vi "testSendCmdStatusServersAandB.vi"(8 "error in (no error)":errorcluster) -> (0 "error out":errorcluster)   [LabVIEW 2018]
doc: "Test the sendCmdStatus.vi in TCP/IP servers A and B."
uses:
  src/TcpServer/TcpServer.lvclass
  src/TcpServer/TcpServer.lvclass/TcpServer.ctl
  src/TcpServerCmd/TcpServerCmd.lvclass/TcpServerCmd.ctl
  <vilib>/addons/_JKI Toolkits/Caraya/classes/Assert/Assert Equal Value_Variant.vi
  src/TcpServerCmd/TcpServerCmd.lvclass
  <vilib>/addons/_JKI Toolkits/Caraya/classes/Test/Test.lvclass
  <vilib>/addons/_JKI Toolkits/Caraya/classes/Assert/Assert.lvclass
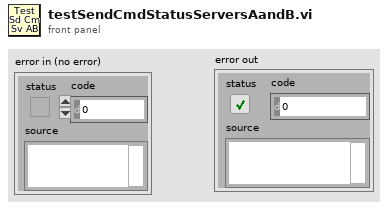
[diagram p1: front panel]
types:
  T1 = typedef "TcpServerCmd.lvclass/userEventTypeDef.ctl" = cluster{"CmdRead":refnum<user-event>, "CmdWrite":refnum<user-event>, "EvtRead":refnum<user-event>, "EvtWrite":refnum<user-event>}
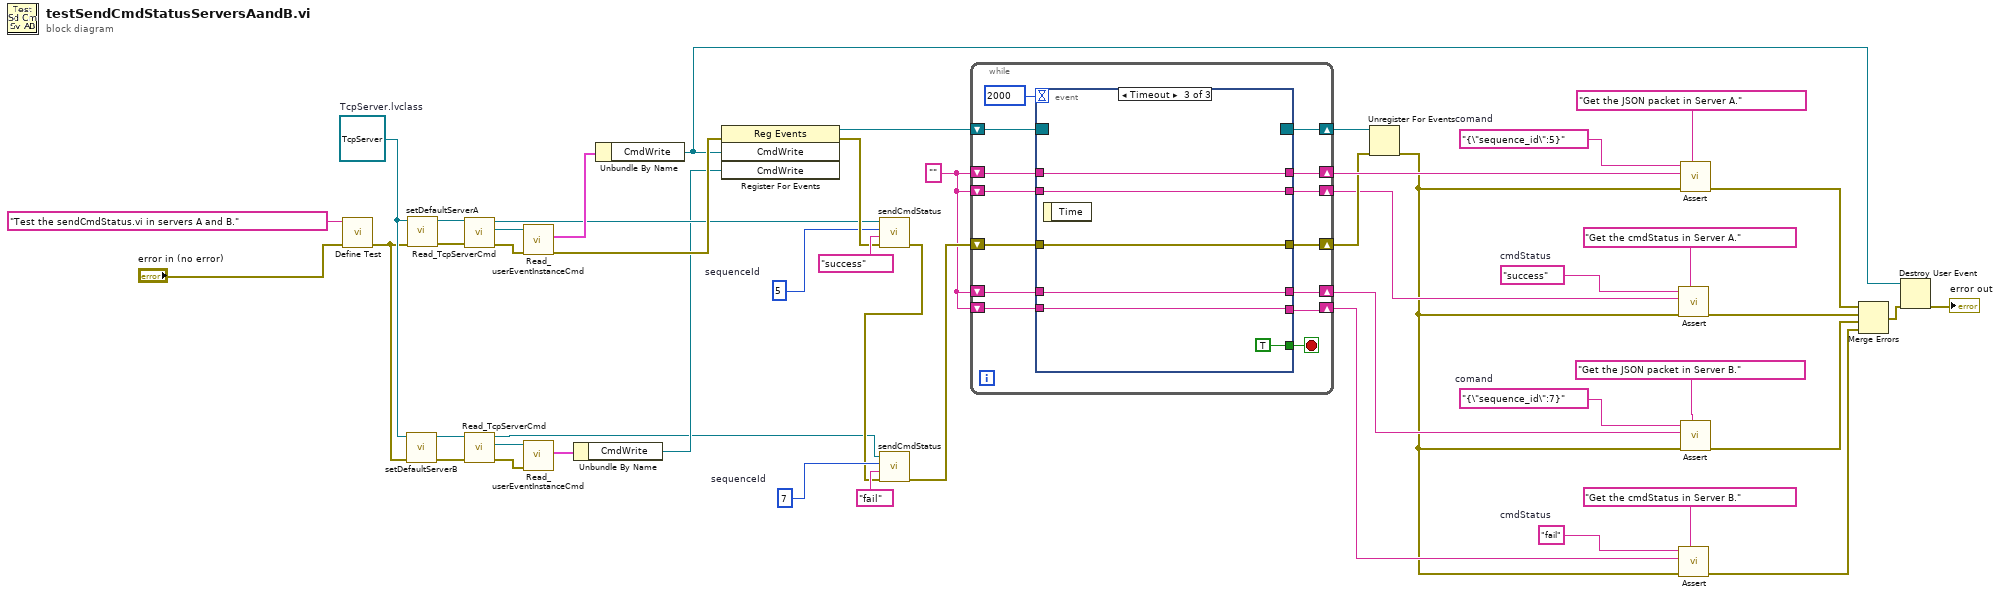
[diagram p0: block diagram]
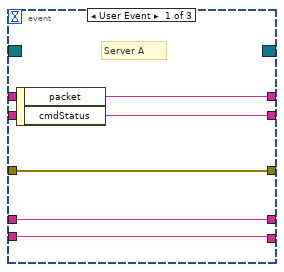
[diagram p2: hidden frame]
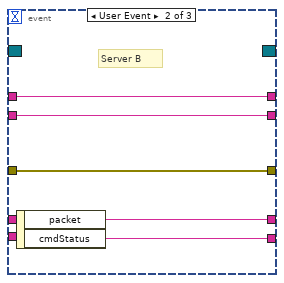
[diagram p3: hidden frame]
diagram:
  w6 = "" ("packet")
  w9 = "fail"  # cmdStatus
  w8 = "{\"sequence_id\":7}"  # comand
  w15 = 7  # sequenceId
  w26 = 5  # sequenceId
  w33 = "success"  # cmdStatus
  w42 = "{\"sequence_id\":5}"  # comand
  w23 = refnum<class "TcpServer.lvclass"> refnum  # TcpServer.lvclass
  n1 = call <vilib>:"Define Test.vi"("error in (no error)"="error in (no error)", "Label (VI Title)"="Test the sendCmdStatus.vi in servers A and B.") -> ("error out"=w22:errorcluster)  [unwired: 9 in]
  n2 = call "setDefaultServerB.vi"("error in (no error)"=w22, "TcpServer.lvclass"=w23) -> ("error out"=w18:errorcluster, "tcpServer out"=w19:refnum<class "TcpServer.lvclass">)  [unwired: 8 in]
  n3 = call "setDefaultServerA.vi"("error in (no error)"=w22, "TcpServer.lvclass"=w23) -> ("error out"=w25:errorcluster, "tcpServer out"=w24:refnum<class "TcpServer.lvclass">)  [unwired: 8 in]
  n4 = call "Read_TcpServerCmd.vi"("error in (no error)"=w25, "TcpServer in"=w24) -> ("error out"=w36:errorcluster, "TcpServerCmd.lvclass"=w37:refnum<class "TcpServerCmd.lvclass">, "TcpServer out"=w28:refnum<class "TcpServer.lvclass">)  [unwired: 7 in]
  n5 = call "Read_TcpServerCmd.vi"("error in (no error)"=w18, "TcpServer in"=w19) -> ("error out"=w21:errorcluster, "TcpServerCmd.lvclass"=w20:refnum<class "TcpServerCmd.lvclass">, "TcpServer out"=w11:refnum<class "TcpServer.lvclass">)  [unwired: 7 in]
  n6 = call "Read_userEventInstanceCmd.vi"("error in (no error)"=w36, "TcpServerCmd in"=w37) -> ("error out"=w35:errorcluster, "userEventInstance"=w34:T1)  [unwired: 7 in, 1 out]
  n7 = call "Read_userEventInstanceCmd.vi"("error in (no error)"=w21, "TcpServerCmd in"=w20) -> ("userEventInstance"=w17:T1)  [unwired: 7 in, 2 out]
  n8 = Unbundle By Name(w17) -> ("CmdWrite"=w16:refnum<user-event>)
  n9 = Unbundle By Name(w34) -> ("CmdWrite"=w27:refnum<user-event>)
  n10 = register-events(error in=w35, w27, w16) -> (reference out=w46:refnum<event-registration>, error out=w45:errorcluster)  [unwired: 1 in]
  n11 = call "sendCmdStatus.vi"("error in (no error)"=w45, "cmdStatus"="success", "sequenceId"=w26, "tcpServer in"=w28) -> ("error out"=w13:errorcluster)  [unwired: 6 in, 1 out]
  n12 = call "sendCmdStatus.vi"("error in (no error)"=w13, "cmdStatus"="fail", "sequenceId"=w15, "tcpServer in"=w11) -> ("error out"=w12:errorcluster)  [unwired: 6 in, 1 out]
  n13 = while {
    shift-right: [w60] -> w40
    shift-left: w46 -> [w63]
    shift-right: [w59] -> w39
    shift-left: w12 -> [w61]
    shift-right: [w62] -> w43
    shift-left: w6 -> [w55]
    shift-right: [w58] -> w31
    shift-left: w6 -> [w54]
    shift-right: [w53] -> w5
    shift-left: w6 -> [w51]
    shift-right: [w52] -> w4
    shift-left: w6 -> [w50]
    stop <- w56 stop-if-true
    n14 = event shown="[2] Timeout" {
      selector: w63 -> [_ _ _]
      dyn-events: [_ _ _] -> w60
      timeout: 2000 -> [_ _ _]
      tunnel: [w68 w70 w77] -> w62
      tunnel: w61 -> [w67 w73 w79]
      tunnel: [w67 w73 w79] -> w59
      tunnel: [w66 w69 w76] -> w58
      tunnel: [w65 w72 w75] -> w53
      tunnel: [w64 w71 w74] -> w52
      tunnel: [_ _ TRUE] -> w56
      tunnel: w55 -> [_ w70 w77]
      tunnel: w54 -> [_ w69 w76]
      tunnel: w51 -> [w65 _ w75]
      tunnel: w50 -> [w64 _ w74]
      event User Event {
        # "Server A"
        n15 = event-data() -> ("packet"=w68:string, "cmdStatus"=w66:string)  [unwired: 1 in]
      }
      event User Event {
        # "Server B"
        n16 = event-data() -> ("packet"=w72:string, "cmdStatus"=w71:string)  [unwired: 1 in]
      }
      event Timeout {
        n17 = event-data() -> ()  [unwired: 1 in, 1 out]
      }
    }
  }
  n18 = Unregister For Events(event registration refnum=w40, error in=w39) -> (error out=w3:errorcluster)
  n19 = call-poly <vilib>:"Assert.vi"("Label"="Get the cmdStatus in Server A.", "error in (no error)"=w3, "Y"=w31, "X"=w33) -> ("error out"=w29:errorcluster)  [unwired: 7 in]
  n20 = call-poly <vilib>:"Assert.vi"("Label"="Get the cmdStatus in Server B.", "error in (no error)"=w3, "Y"=w4, "X"=w9) -> ("error out"=w1:errorcluster)  [unwired: 7 in]
  n21 = call-poly <vilib>:"Assert.vi"("Label"="Get the JSON packet in Server A.", "error in (no error)"=w3, "Y"=w43, "X"=w42) -> ("error out"=w41:errorcluster)  [unwired: 7 in]
  n22 = call-poly <vilib>:"Assert.vi"("Label"="Get the JSON packet in Server B.", "error in (no error)"=w3, "Y"=w5, "X"=w8) -> ("error out"=w2:errorcluster)  [unwired: 7 in]
  n23 = Merge Errors(w41, w29, w2, w1) -> (w30:errorcluster)
  n24 = Destroy User Event(user event=w27, error in=w30) -> (error out=→"error out":errorcluster)
